vi "Return Run VI State.vi"(8 "error in (no error)":errorcluster, 9 "Error From Run VI":errorcluster, 10 "Indicators":refnum<class "tBSONDocument.lvclass">, 11 "tWorkerTCPConnection in":refnum<class "tWorkerTCPConnection.lvclass">) -> (0 "error out":errorcluster, 3 "tWorkerTCPConnection out":refnum<class "tWorkerTCPConnection.lvclass">)   [LabVIEW 2014, in "tWorkerTCPConnection.lvlib" / "tWorkerTCPConnection.lvclass"]
uses:
  tWorkerTCPConnection.lvclass
  BSON/tBSONDocument/tBSONDocument.lvclass
  <vilib>/ActorFramework/Actor/Actor.lvclass/Actor.ctl
  <vilib>/ActorFramework/Message Enqueuer/Message Enqueuer.lvclass/Message Enqueuer.ctl
  msgs/Send Message Msg/Send Message Msg.lvclass/Send Message Msg.ctl
  <vilib>/ActorFramework/Message Enqueuer/Init from Existing Queue.vi
  <vilib>/ActorFramework/Message Enqueuer/Enqueue.vi
  BSON/tBSONDocument/addBooleanElement.vi
  BSON/tBSONDocument/addI32Element.vi
  BSON/tBSONDocument/addStringElement.vi
  <vilib>/ActorFramework/Message Priority Queue/Priority Enqueue.vi
  <vilib>/ActorFramework/Message Enqueuer/Message Enqueuer.lvclass
  msgs/Send Message Msg/Send Message Msg.lvclass
  <vilib>/ActorFramework/Actor/Actor.lvclass
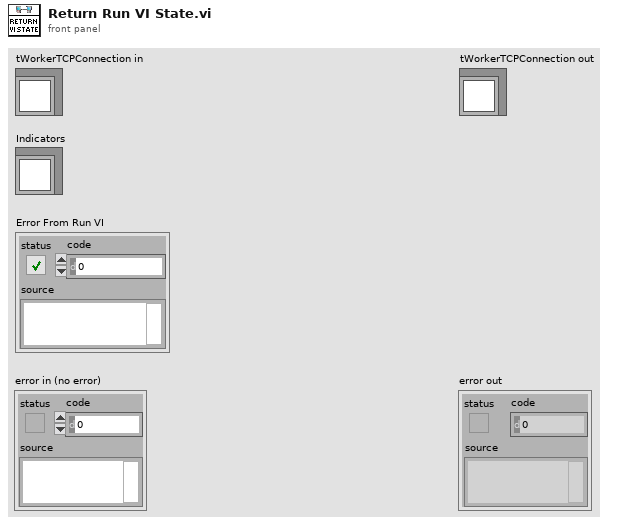
[diagram p1: front panel]
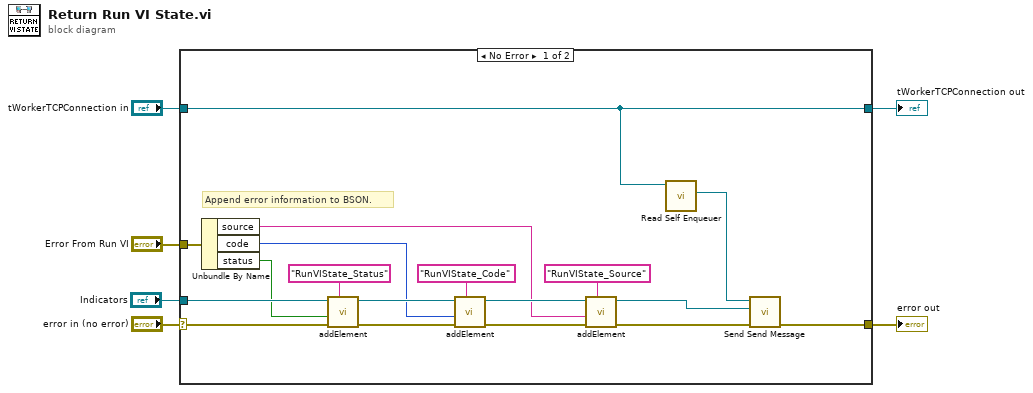
[diagram p0: block diagram]
diagram:
  n1 = case shown="No Error" "error in (no error)" {
    selector: "error in (no error)" -> [w24 w26]
    tunnel: [w7 w26] -> w5
    tunnel: [w11 w25] -> w3
    tunnel: "tWorkerTCPConnection in" -> [w11 w25]
    tunnel: "Indicators" -> [w22 _]
    tunnel: "Error From Run VI" -> [w21 _]
    frame No Error {
      # "Append error information to BSON."
      n2 = Unbundle By Name(w21) -> ("source"=w12:string, "code"=w13:i32, "status"=w20:bool)
      n3 = call-poly "addElement.vi"("Name"="RunVIState_Status", "error in (no error)"=w24, "Value"=w20, "tBSONDocument in"=w22) -> ("error out"=w14:errorcluster, "tBSONDocument out"=w18:refnum<class "tBSONDocument.lvclass">)  [unwired: 6 in]
      n4 = call-poly "addElement.vi"("Name"="RunVIState_Code", "error in (no error)"=w14, "Value"=w13, "tBSONDocument in"=w18) -> ("error out"=w15:errorcluster, "tBSONDocument out"=w16:refnum<class "tBSONDocument.lvclass">)  [unwired: 6 in]
      n5 = call-poly "addElement.vi"("Name"="RunVIState_Source", "error in (no error)"=w15, "Value"=w12, "tBSONDocument in"=w16) -> ("error out"=w8:errorcluster, "tBSONDocument out"=w9:refnum<class "tBSONDocument.lvclass">)  [unwired: 6 in]
      n6 = call <vilib>:"Read Self Enqueuer.vi"("Actor"=w11) -> ("Self Enqueuer"=w10:refnum<class "Message Enqueuer.lvclass">)  [unwired: 10 in]
      n7 = call "Send Send Message.vi"("error in (no error)"=w8, "Message"=w9, "Message Enqueuer"=w10) -> ("error out"=w7:errorcluster)  [unwired: 7 in, 1 out]
    }
    frame Error {
    }
  }
  "error out" <- w5
  "tWorkerTCPConnection out" <- w3
